vi "Untitled 1.vi"() -> ()   [LabVIEW 2017]
uses:
  <vilib>/ethernetip/ethernetip.llb/ethernetip.ctl
  <vilib>/ethernetip/ethernetip.llb/EthernetIP SLC500 Read Integer.vi
  <vilib>/ethernetip/ethernetip.lvlib
panel:
  out "error out":errorcluster
  out "Data":i16[](array[numeric])
  out "Session out":T1
  in  "error in":errorcluster
  in  "Number of Elements":u32=1
  in  "Element Number":u16
  in  "Network Path":string
  in  "Timeout (ms)":i32=1000
  in  "File Number":u16=7
  in  "Session in":T1="Default"
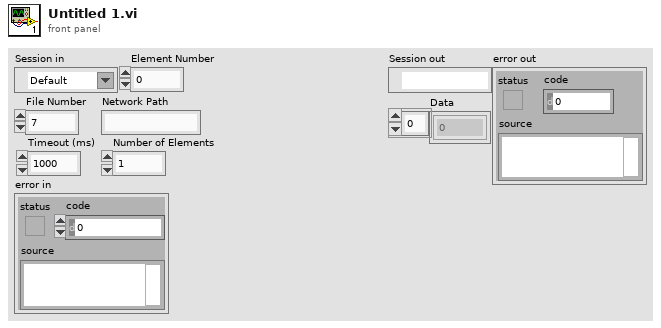
[diagram p1: front panel]
types:
  T1 = typedef "ethernetip.lvlib/ethernetip.ctl" = refnum<k21>
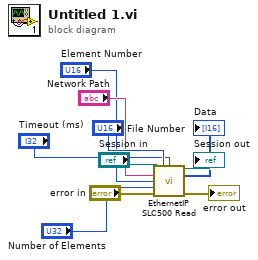
[diagram p0: block diagram]
diagram:
  n1 = call-poly <vilib>:"EthernetIP SLC500 Read.vi"("Session in"="Session in", "File Number"="File Number", "Timeout (ms)"="Timeout (ms)", "Network Path"="Network Path", "Element Number"="Element Number", "Number of Elements"="Number of Elements", "error in"="error in") -> ("Session out"=→"Session out":T1, "Data"=→"Data":i16[], "error out"=→"error out":errorcluster)  [unwired: 6 in]
